vi "Cut start datum.vi"(3 "bytestream":refnum<class "Bytestream.lvclass">) -> (0 "data":u8[](array[numeric]) format="%02x", 1 "bytestream out":refnum<class "Bytestream.lvclass">)   [LabVIEW 2020, in "NI_Bytestream.lvlib" / "Bytestream.lvclass"]
uses:
  <vilib>/Array/Bytestream/Bytestream.lvclass
  <vilib>/Array/Bytestream/Bytestream.lvclass/Bytestream.ctl
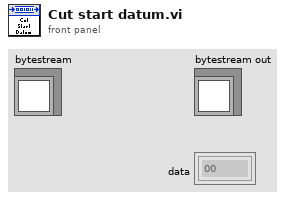
[diagram p1: front panel]
types:
  T1 = typedef "NI_Bytestream.lvlib/Bytestream.lvclass/Datum.ctl" = cluster{"array":u8[], "index":i32}
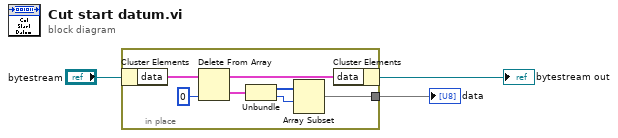
[diagram p0: block diagram]
diagram:
  n1 = in-place {
    in-place-border: [w4] -> w2
    n2 = in-place-cluster #1("bytestream") -> ("data"=w10:T1[])
    n3 = Delete From Array(array=w10, index=0) -> (deleted portion=w7:T1, array with subset deleted=w8:T1[])  [unwired: 1 in]
    n4 = Unbundle(w7) -> ("array"=w6:u8[], "index"=w5:i32)
    n5 = Array Subset(array=w6, index=w5) -> (w4:u8[])  [unwired: 1 in]
    n6 = in-place-cluster #1("data"=w8) -> (→"bytestream out":refnum<class "Bytestream.lvclass">)
  }
  "data" <- w2
